vi "rad_Configure Individual BlacklistSettings Dialog.vi"(8 "error in (no error)":errorcluster, 11 "blacklistObject In":T1) -> (0 "error out":errorcluster, 2 "Canceled":bool, 3 "blacklistObject Out":T1)   [LabVIEW 2014]
uses:
  Util/FP Control/FP Control Functions.ctl
  TypeDefs/rad_Blacklist Object.ctl
panel:
  in  "Blacklist During Deployment":bool
  in  "File Path or Directory":string
  in  "Blacklist During Retrieval":bool
  in  "Cancel":bool
  in  "OK":bool
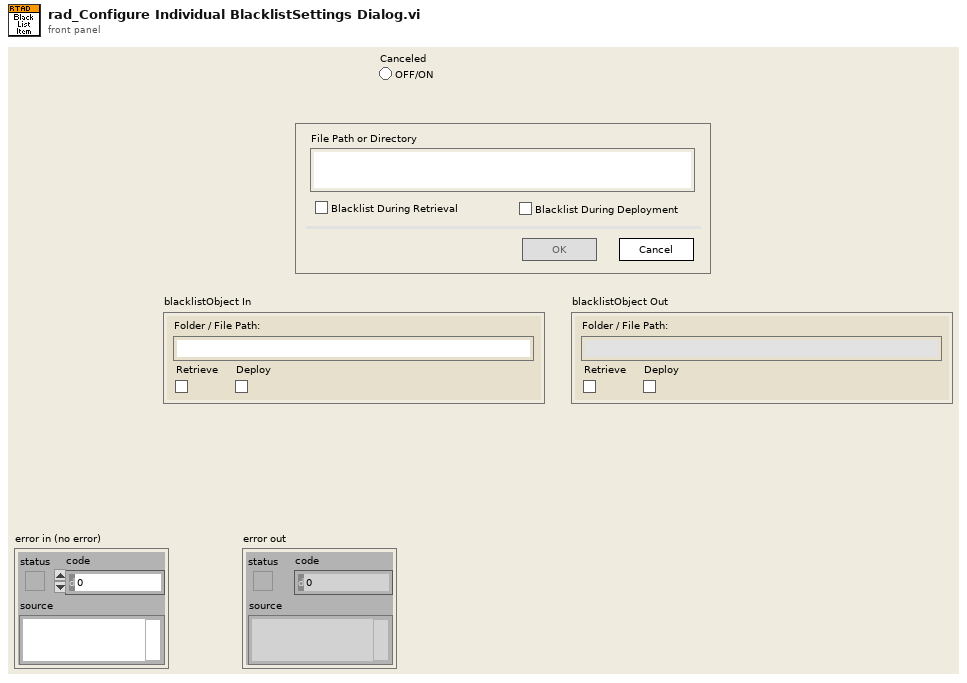
[diagram p1: front panel]
types:
  T1 = typedef "rad_Blacklist Object.ctl" = cluster{"Folder / File Path:":string, "Retrieve":bool, "Deploy":bool}
  T2 = typedef "FP Control Functions.ctl" = enum16{"Open", "Close", "Bring To Front", "Center"}
  T3 = enum8{"Enabled", "Disabled", "Disabled and Grayed Out"}
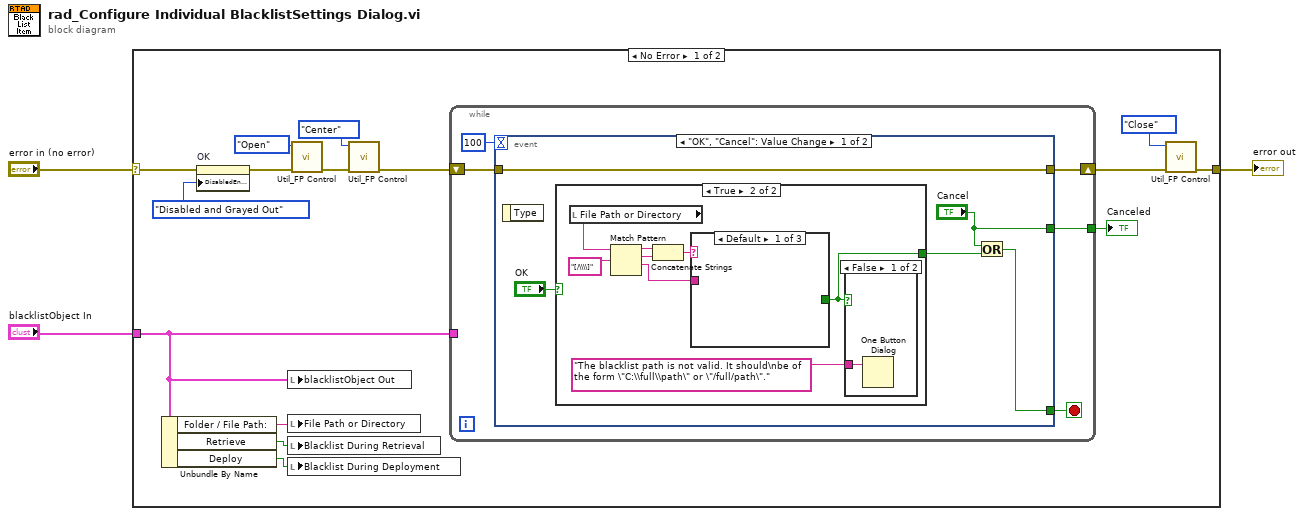
[diagram p0: block diagram]
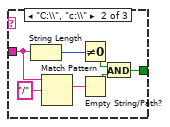
[diagram p4: hidden frame]
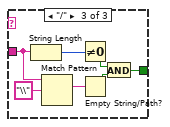
[diagram p5: hidden frame]
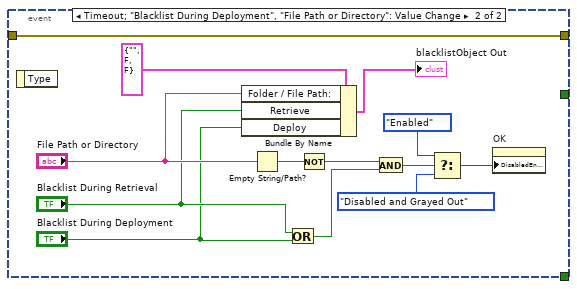
[diagram p6: hidden frame]
diagram:
  n1 = case shown="No Error" "error in (no error)" {
    selector: "error in (no error)" -> [w8 w65]
    tunnel: [w11 w65] -> w3
    tunnel: "blacklistObject In" -> [w4 _]
    frame No Error {
      n2 = Unbundle By Name(w4) -> ("Folder / File Path:"=w7:string, "Retrieve"=w6:bool, "Deploy"=w5:bool)
      n3 = property on="OK" class="Bool"(error in=w8, "DisabledEnum"=T3."Disabled and Grayed Out" ("Disabled")) -> (error out=w15:errorcluster)  [unwired: 1 in, 1 out]
      n4 = local write "blacklistObject Out"(w4) -> ()
      n5 = local write "File Path or Directory"(w7) -> ()
      n6 = local write "Blacklist During Retrieval"(w6) -> ()
      n7 = local write "Blacklist During Deployment"(w5) -> ()
      n8 = call "Util_FP Control.vi"("error in (no error)"=w15, "Function"=FP_Control_Functions."Open") -> ("error out"=w14:errorcluster)  [unwired: 9 out]
      n9 = call "Util_FP Control.vi"("error in (no error)"=w14, "Function"=FP_Control_Functions."Center") -> ("error out"=w16:errorcluster)  [unwired: 9 out]
      n10 = while {
        tunnel: [w22] -> w10
        shift-right: [w20] -> w12
        shift-left: w16 -> [w21]
        tunnel: w4 -> [_]
        stop <- w23 stop-if-true
        n11 = event shown="[0] \"OK\", \"Cancel\": Value Change" {
          selector: _ -> [_ _]
          dyn-events: _ -> [_ _]
          timeout: 100 -> [_ _]
          tunnel: [w28 _] -> w23
          tunnel: ["Cancel" _] -> w22
          tunnel: w21 -> [w26 w52]
          tunnel: [w26 w52] -> w20
          event "OK", "Cancel": Value Change {
            n12 = event-data() -> ()  [unwired: 1 in, 1 out]
            n13 = case shown="True" "OK" {
              tunnel: [_ w30] -> w24
              frame False {
              }
              frame True {
                n14 = local read "File Path or Directory"() -> (w36:string)
                n15 = Match Pattern(string=w36, regular expression="[/\\\\]") -> (before substring=w33:string, match substring=w34:string, after substring=w31:string)  [unwired: 1 in, 1 out]
                n16 = Concatenate Strings(w33, w34) -> (w32:string)
                n17 = case shown="Default" w32 {
                  tunnel: w31 -> [_ w44 w51]
                  tunnel: [_ w38 w45] -> w30
                  frame Default {
                  }
                  frame "C:\\", "c:\\" {
                    n18 = String Length(string=w44) -> (length=w42:i32)
                    n19 = Match Pattern(string=w44, regular expression="/") -> (match substring=w41:string)  [unwired: 1 in, 3 out]
                    n20 = Not Equal To 0?(x=w42) -> (x != 0?=w40:bool)
                    n21 = Empty String/Path?(string/path=w41) -> (empty?=w39:bool)
                    n22 = And(x=w40, y=w39) -> (x .and. y?=w38:bool)
                  }
                  frame "/" {
                    n23 = String Length(string=w51) -> (length=w49:i32)
                    n24 = Match Pattern(string=w51, regular expression="\\") -> (match substring=w48:string)  [unwired: 1 in, 3 out]
                    n25 = Not Equal To 0?(x=w49) -> (x != 0?=w47:bool)
                    n26 = Empty String/Path?(string/path=w48) -> (empty?=w46:bool)
                    n27 = And(x=w47, y=w46) -> (x .and. y?=w45:bool)
                  }
                }
                n28 = case shown="False" w30 {
                  tunnel: "The blacklist path is not valid. It should\nbe of the form \"C:\\full\\path\" or \"/full/path\"." -> [w37 _]
                  frame False {
                    n29 = One Button Dialog(message=w37) -> ()  [unwired: 1 in, 1 out]
                  }
                  frame True {
                  }
                }
              }
            }
            n30 = Or(x="Cancel", y=w24) -> (x .or. y?=w28:bool)
          }
          event Timeout; "Blacklist During Deployment", "File Path or Directory": Value Change {
            n31 = event-data() -> ()  [unwired: 1 in, 1 out]
            n32 = Bundle By Name(cluster=T1 {"Folder / File Path:"="", "Retrieve"=FALSE, "Deploy"=FALSE} ("blacklistObject In"), "Folder / File Path:"="File Path or Directory", "Retrieve"="Blacklist During Retrieval", "Deploy"="Blacklist During Deployment") -> (→"blacklistObject Out":T1)
            n33 = Empty String/Path?(string/path="File Path or Directory") -> (empty?=w64:bool)
            n34 = Or(x="Blacklist During Retrieval", y="Blacklist During Deployment") -> (x .or. y?=w62:bool)
            n35 = Not(x=w64) -> (.not. x?=w63:bool)
            n36 = And(x=w63, y=w62) -> (x .and. y?=w61:bool)
            n37 = Select(t=T3."Enabled" ("Disabled"), s=w61, f=T3."Disabled and Grayed Out" ("Disabled")) -> (s? t:f=w58:T3)
            n38 = property on="OK" class="Bool"("DisabledEnum"=w58) -> ()  [unwired: 2 in, 2 out]
          }
        }
      }
      "Canceled" <- w10
      n39 = call "Util_FP Control.vi"("error in (no error)"=w12, "Function"=FP_Control_Functions."Close") -> ("error out"=w11:errorcluster)  [unwired: 9 out]
    }
    frame Error {
    }
  }
  "error out" <- w3
